vi "String to Boolean.vi"(1 "Default(F)":bool, 3 "String":string) -> (0 "Boolean":bool)   [LabVIEW 2017]
doc: "Converts a string to a boolean from a recognised word list: values such as 1, Active, True, On and Valid give TRUE, while 0, Inactive, False, Off and Invalid give FALSE. Leading and trailing whitespace is trimmed and matching is case-insensitive. Any other string returns the Default(F) value."
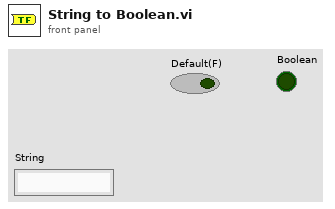
[diagram p1: front panel]
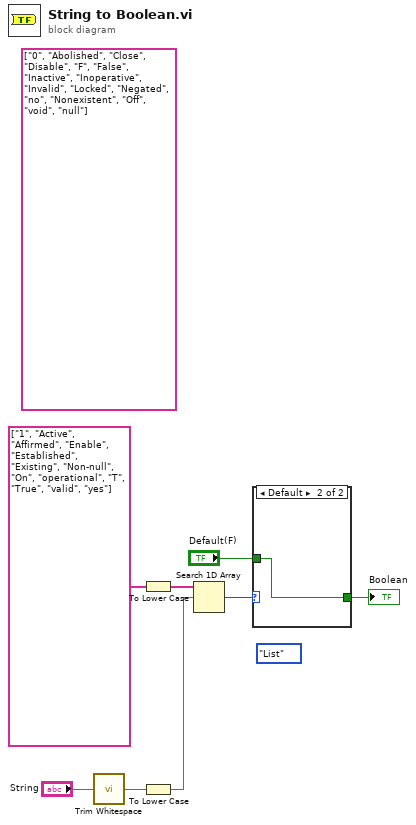
[diagram p0: block diagram]
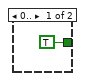
[diagram p2: hidden frame]
diagram:
  (unwired) string[] ["0", "Abolished", "Close", "Disable", "F", "False", "Inactive", "Inoperative", "Invalid", "Locked", "Negated", "no", "Nonexistent", "Off", "void", "null"]
  (unwired) enum16{"List", "Add", "Remove"}."List" ("Enum")
  n1 = call <vilib>:"Trim Whitespace.vi"("string"="String") -> ("trimmed string"=w1:string)  [unwired: 1 in]
  n2 = To Lower Case(string=string[] ["1", "Active", "Affirmed", "Enable", "Established", "Existing", "Non-null", "On", "operational", "T", "True", "valid", "yes"]) -> (all lower case string=w5:string[])
  n3 = To Lower Case(string=w1) -> (all lower case string=w3:string)
  n4 = Search 1D Array(1D array=w5, element=w3) -> (index of element=w2:i32)  [unwired: 1 in]
  n5 = case shown="Default" w2 {
    tunnel: [TRUE w10] -> w6
    tunnel: "Default(F)" -> [_ w10]
    frame 0.. {
    }
    frame Default {
    }
  }
  "Boolean" <- w6
